vi "总氮固定站质控流程.vi"(6 "队列输入TN":refnum<queue>, 9 "总氮":bool, 10 "总氮量程切换":enum32{"H", "L", "AUTO"}(ring)=enum."AUTO") -> (3 "布尔":bool)   [LabVIEW 2016, in "质控单元.lvlib"]
panel:
  out "总氮中断报警":bool
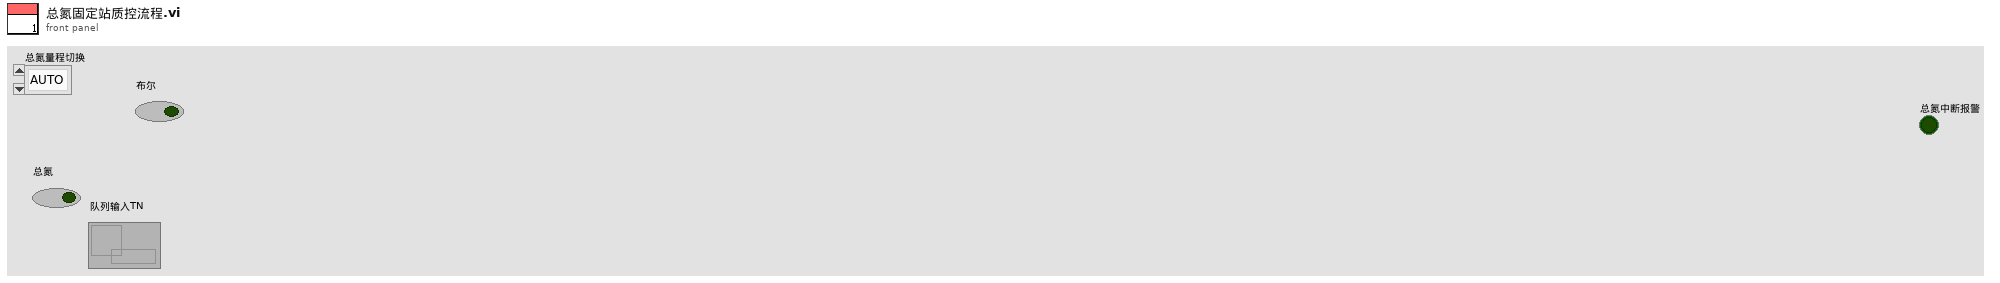
[diagram p1: front panel]
types:
  T1 = enum16{"待机", "启动氨氮水样", "氨氮测量中", "启动氨氮加标", "启动氨氮加标回收", "氨氮加标回收测量中", "启动总氮水样", "总氮测量中", "启动总氮加标", "启动总氮加标回收", "总氮加标回收测量中", "启动总磷水样", "总磷水样测量中", "启动总磷加标", "启动总磷加标回收", "总磷加标回收测量中", "结束"}
  T2 = cluster{"站号":u16, "量程切换":enum32{"H", "L", "AUTO"}, "控制命令":enum16{"启动测量", "标样核查", "零点核查", "跨度核查", "空白测试", "平行样测试", "加标回收", "空白校准", "标样校准", "初始化（清洗）", "停止测试", "仪器重启", "校时", "模式设置", "测量间隔设置"}, "模式设置":enum16{"待机", "连续模式", "周期模式", "定点模式", "受控模式", "手动模式"}, "测量间隔":u16}
  T3 = cluster{"时间标识":timestamp, "设备":string, "日志信息":string}
  T4 = cluster{"系统时间":timestamp, "工作状态":enum16{"空闲", "水样测试", "标样核查", "零点核查", "跨度核查", "空白测试", "平行样测试", "加标回收", "空白校准", "标样校准", "初始化（清洗）"}, "测量模式":enum16{"待机", "连续模式", "周期模式", "定点模式", "受控模式", "手动模式"}, "告警代码":enum16{"无告警", "缺试剂告警", "缺水样告警", "缺蒸馏水告警", "缺标液告警", "仪表漏液告警", "标定异常告警", "超量程告警", "加热异常", "低试剂预警", "超上限告警", "超下限告警", "仪表内部其他异常", "滴定异常告警", "电极异常告警", "量程切换告警", "参数设置告警", "PH电极电位异常", "电导率电极异常", "浊度光度异常", "溶解氧电极异常", "溶解氧光强异常", "温度异常告警", "PH异常告警", "溶解氧异常告警", "电导率异常告警", "浊度异常告警", "叶绿素异常告警", "藻密度异常告警", "蓝绿藻异常告警", "ORP异常告警", "氨氮异常告警", "清洁刷异常告警", "SD卡异常告警", "蓝牙异常告警", "Wifi异常告警", "流程异常告警"}, "故障代码":enum16{"无故障", "电机故障", "温度故障", "通讯故障", "滴定故障"}, "日志代码":u16, "软件版本":u16, "F0":sgl, "F1":sgl, "F2":sgl, "F3":sgl, "T":sgl, "H":sgl, "id":u16, "flowid":u16, "量程":u16, "总磷控温温度1":sgl, "营养盐控温温度2":sgl, "ADC":sgl}
  T5 = enum16{"空闲", "水样测试", "标样核查", "零点核查", "跨度核查", "空白测试", "平行样测试", "加标回收", "空白校准", "标样校准", "初始化（清洗）"}
  T6 = cluster{"因子编码":u32, "单位":u16, "标样参考值":sgl, "水样数据时间":timestamp, "水样实测值":sgl, "水样数据标识":string, "标样数据时间":timestamp, "标样实测值":sgl, "标样数据标识":string, "空白数据时间":timestamp, "空白实测值":sgl, "空白数据标识":string, "零点核查数据时间":timestamp, "零点核查实测值":sgl, "零点核查数据标识":string, "跨度核查数据时间":timestamp, "跨度核查实测值":sgl, "跨度核查数据标识":string, "加标回收数据时间":timestamp, "加标回收实测值":sgl, "加标回收数据标识":string, "平行样数据时间":timestamp, "平行样实测值":sgl, "平行样数据标识":string}
  T7 = cluster{"量程":dbl, "检出限":dbl, "加标前水样浓度":dbl, "加标后水样浓度":dbl, "加标水杯定容体积":dbl, "加标母液浓度":dbl, "加标体积":dbl, "加标回收率":dbl}
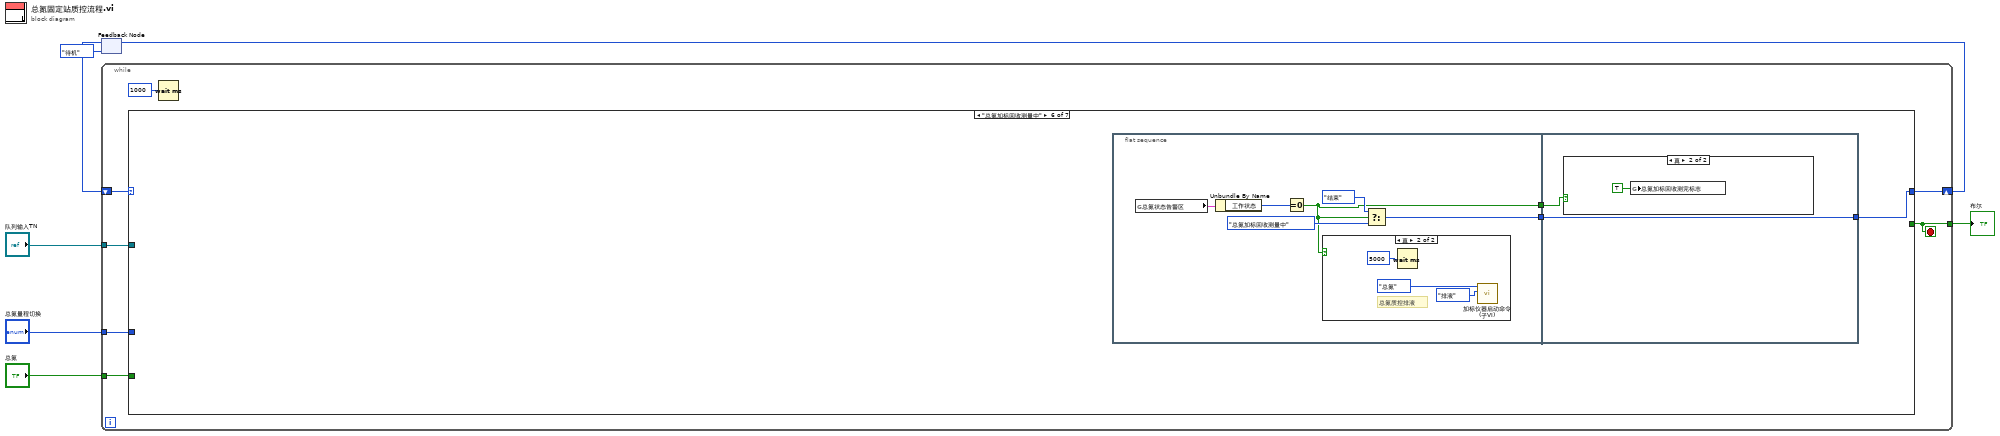
[diagram p0: block diagram]
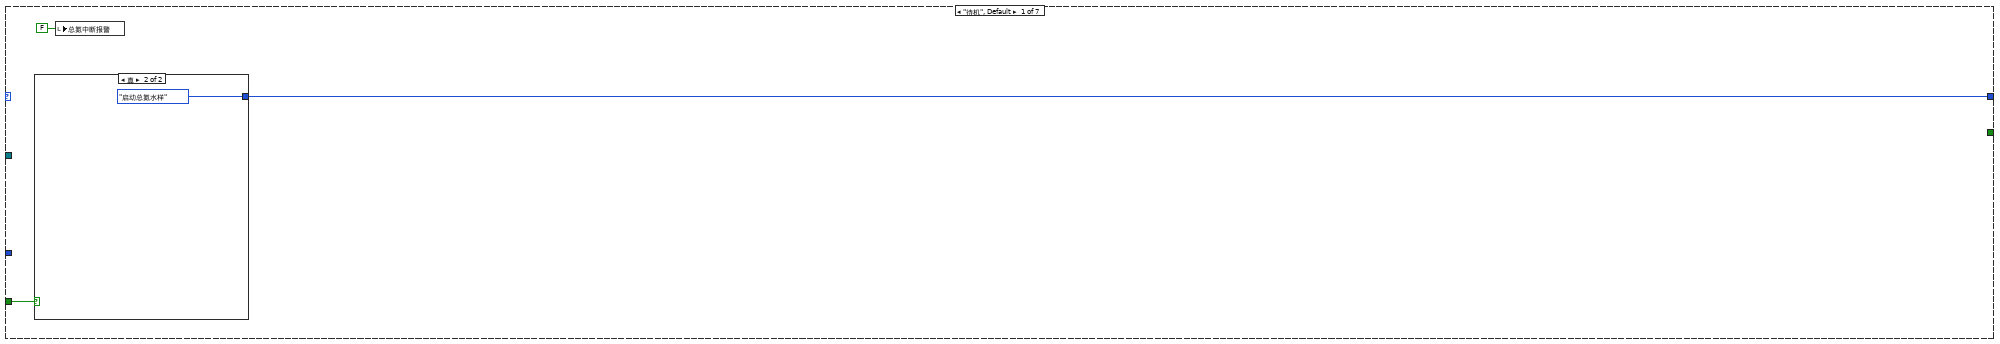
[diagram p2: hidden frame]
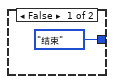
[diagram p3: hidden frame]
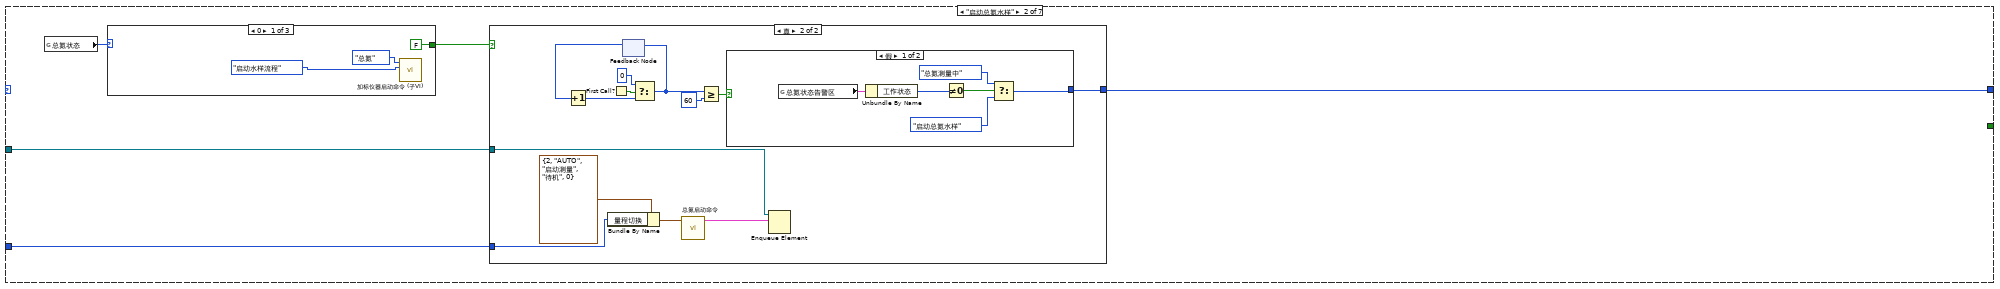
[diagram p4: hidden frame]
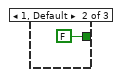
[diagram p5: hidden frame]
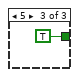
[diagram p6: hidden frame]
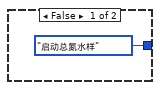
[diagram p7: hidden frame]
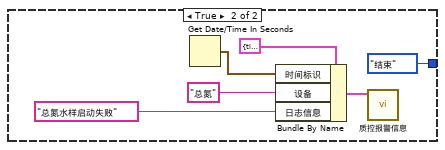
[diagram p8: hidden frame]
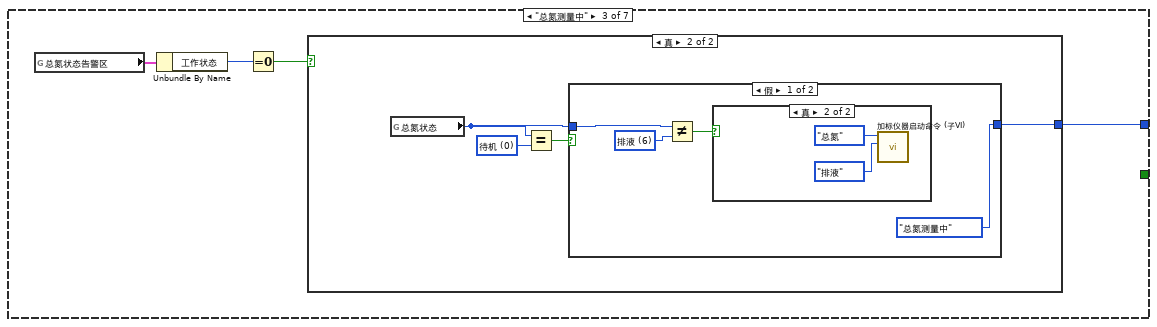
[diagram p9: hidden frame]
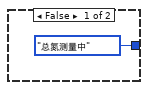
[diagram p10: hidden frame]
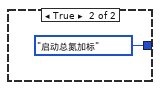
[diagram p12: hidden frame]
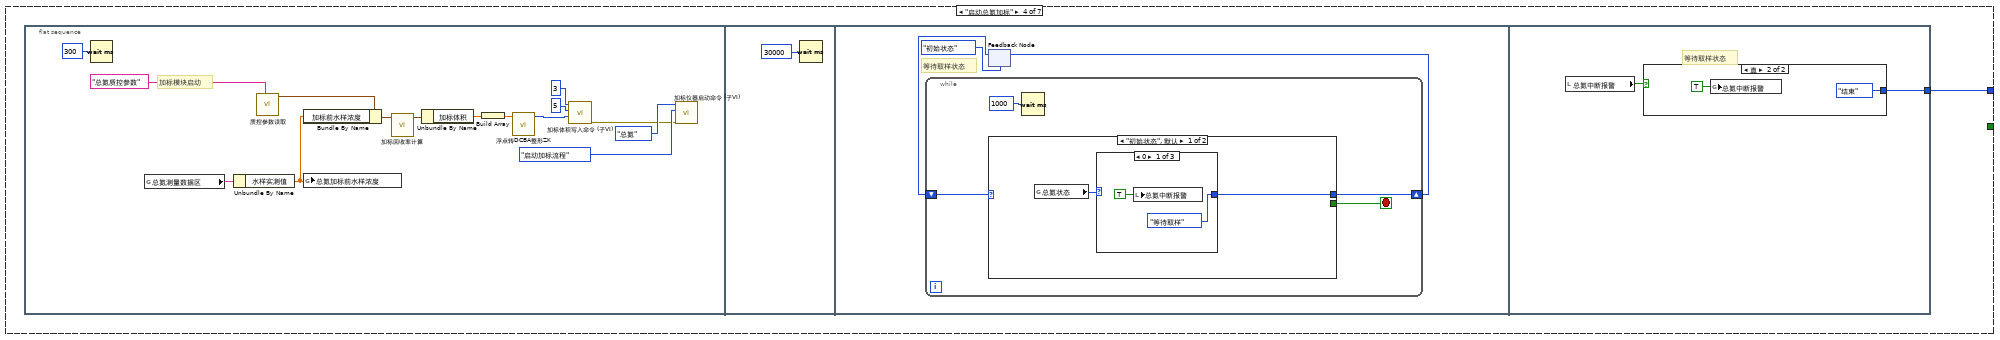
[diagram p13: hidden frame]
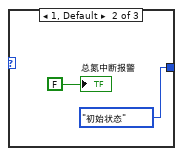
[diagram p14: hidden frame]
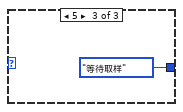
[diagram p15: hidden frame]
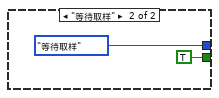
[diagram p16: hidden frame]
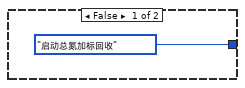
[diagram p17: hidden frame]
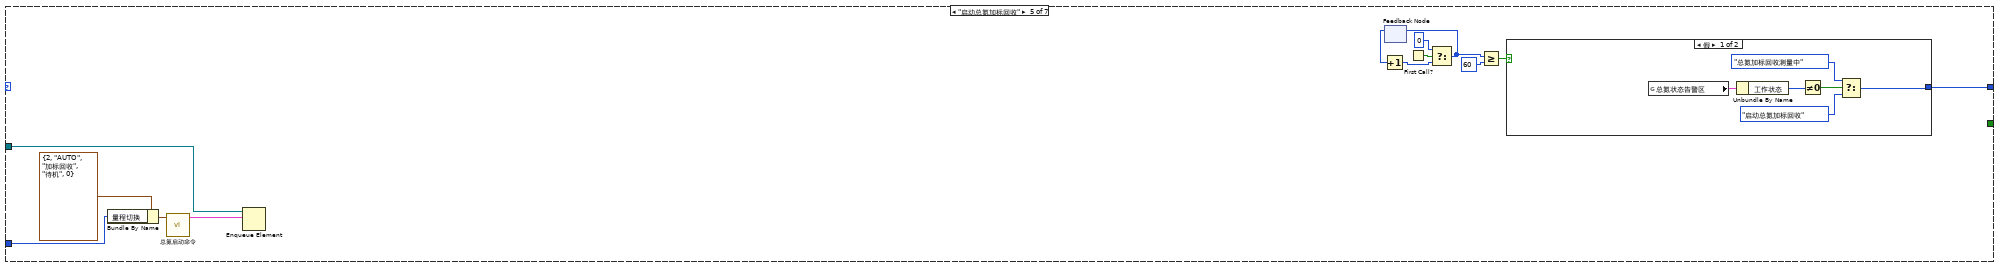
[diagram p18: hidden frame]
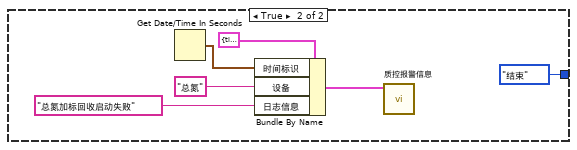
[diagram p19: hidden frame]
diagram:
  n1 = feedback #1(T1."待机") -> (w1:T1)
  n2 = while {
    tunnel: "队列输入TN" -> [w12]
    tunnel: "总氮量程切换" -> [w11]
    tunnel: "总氮" -> [w14]
    tunnel: [w8] -> w6
    shift-right: [w13] -> w4
    shift-left: w1 -> [w10]
    stop <- w8 stop-if-true
    n3 = case shown="\"总氮加标回收测量中\"" w10 {
      tunnel: [w17 w24 w56 w72 w115 w136 T1."结束"] -> w13
      tunnel: [_ _ _ _ _ _ TRUE] -> w8
      tunnel: w14 -> [w16 _ _ _ _ _ _]
      tunnel: w12 -> [_ w23 _ _ w114 _ _]
      tunnel: w11 -> [_ w22 _ _ w111 _ _]
      frame "待机", Default {
        n4 = case shown="真" w16 {
          tunnel: [T1."结束" T1."启动总氮水样"] -> w17
          frame False {
          }
          frame True {
          }
        }
        n5 = local write "总氮中断报警"(FALSE ("氨氮中断报警")) -> ()
      }
      frame "启动总氮水样" {
        n6 = global read "加标回收状态全局变量.vi" "总氮状态"() -> (w21:u16)
        n7 = case shown="0" w21 {
          tunnel: [FALSE ("s") FALSE ("s") TRUE ("s")] -> w20
          frame 0 {
            n8 = call "加标仪器启动命令 (子VI).vi"("启动命令"=enum16{"启动水样流程", "启动加标流程", "排液", "停止"}."启动水样流程", "仪器"=enum16{"", "氨氮", "总磷", "总氮", "CODMn", "CODCr"}."总氮") -> ()  [unwired: 9 in, 1 out]
          }
          frame 1, Default {
          }
          frame 5 {
          }
        }
        n9 = case shown="真" w20 {
          tunnel: [T1."启动总氮水样" w43] -> w24
          tunnel: w23 -> [_ w35]
          tunnel: w22 -> [_ w32]
          frame False {
          }
          frame True {
            n10 = Bundle By Name(cluster=T2 {"站号"=2, "量程切换"=enum."AUTO", "控制命令"=enum."启动测量", "模式设置"=enum."待机", "测量间隔"=0} ("参数"), "量程切换"=w32) -> (w34:T2)
            n11 = First Call?() -> (First Call?: T/F=w41:bool)
            n12 = feedback #2() -> (w40:i32)  [unwired: 1 in]
            n13 = Increment(x=w40) -> (x+1=w39:i32)
            n14 = Select(t=0, s=w41, f=w39) -> (s? t:f=w38:i32)
            n15 = feedback-in #2(w38) -> ()
            n16 = call "总氮启动命令.vi"("参数"=w34) -> ("启动命令"=w31:cluster{"命令":string, "data":variant})  [unwired: 10 in]
            n17 = Greater Or Equal?(x=w38, y=60) -> (x >= y?=w36:bool)
            n18 = case shown="假" w36 {
              tunnel: [w48 T1."结束"] -> w43
              frame False {
                n19 = global read "与总氮交互全局.vi" "总氮状态告警区"() -> (w45:T4)
                n20 = Unbundle By Name(w45) -> ("工作状态"=w44:T5)
                n21 = Not Equal To 0?(x=w44) -> (x != 0?=w49:bool)
                n22 = Select(t=T1."总氮测量中", s=w49, f=T1."启动总氮水样") -> (s? t:f=w48:T1)
              }
              frame True {
                n23 = Get Date/Time In Seconds() -> (seconds since 1Jan1904=w55:timestamp)
                n24 = Bundle By Name(cluster=T3 {"时间标识"=timestamp(0 s since 1904-01-01), "设备"="", "日志信息"=""} ("data in"), "时间标识"=w55, "设备"="总氮", "日志信息"="总氮水样启动失败") -> (w50:T3)
                n25 = call "质控报警信息.vi"("data in"=w50) -> ()  [unwired: 10 in, 1 out]
              }
            }
            n26 = Enqueue Element(queue=w35, element=w31) -> ()  [unwired: 2 in, 3 out]
          }
        }
      }
      frame "总氮测量中" {
        n27 = global read "与总氮交互全局.vi" "总氮状态告警区"() -> (w59:T4)
        n28 = Unbundle By Name(w59) -> ("工作状态"=w57:T5)
        n29 = Equal To 0?(x=w57) -> (x = 0?=w58:bool)
        n30 = case shown="真" w58 {
          tunnel: [T1."总氮测量中" w62] -> w56
          frame False {
          }
          frame True {
            w64 = u16 0 items=["待机", "润洗", "进样", "进样完成", "柱塞泵加标", "等待取液", "排液"] ("氨氮状态")
            n31 = global read "加标回收状态全局变量.vi" "总氮状态"() -> (w61:u16)
            n32 = Equal?(x=w61, y=w64) -> (x = y?=w63:bool)
            n33 = case shown="假" w63 {
              tunnel: [T1."总氮测量中" T1."启动总氮加标"] -> w62
              tunnel: w61 -> [w65 _]
              frame False {
                w67 = u16 6 items=["待机", "润洗", "进样", "进样完成", "柱塞泵加标", "等待取液", "排液"] ("氨氮状态")
                n34 = Not Equal?(x=w65, y=w67) -> (x != y?=w66:bool)
                n35 = case shown="真" w66 {
                  frame False {
                  }
                  frame True {
                    n36 = call "加标仪器启动命令 (子VI).vi"("启动命令"=enum16{"启动水样流程", "启动加标流程", "排液", "停止"}."排液", "仪器"=enum16{"", "氨氮", "总磷", "总氮", "CODMn", "CODCr"}."总氮") -> ()  [unwired: 9 in, 1 out]
                  }
                }
              }
              frame True {
              }
            }
          }
        }
      }
      frame "启动总氮加标" {
        n37 = flat-sequence {
          tunnel: [w106] -> w72
          frame #0 {
            # "加标模块启动"
            n38 = Wait (ms)(milliseconds to wait=u32 300 ("等待时间（毫秒）")) -> ()  [unwired: 1 out]
            n39 = global read "与总氮交互全局.vi" "总氮测量数据区"() -> (w80:T6)
            n40 = Unbundle By Name(w80) -> ("水样实测值"=w82:sgl)
            n41 = call "质控参数读取.vi"("section"="总氮质控参数") -> ("参数"=w85:T7)  [unwired: 9 in, 1 out]
            n42 = Bundle By Name(cluster=w85, "加标前水样浓度"=w82) -> (w86:T7)
            n43 = global write "水样浓度全局.vi" "总氮加标前水样浓度"(w82) -> ()
            n44 = call "加标回收率计算.vi"("参数"=w86) -> ("参数 out"=w84:T7)  [unwired: 9 in, 1 out]
            n45 = Unbundle By Name(w84) -> ("加标体积"=w83:dbl)
            n46 = Build Array(w83) -> (w79:dbl[])
            n47 = call "浮点转DCBA整形ZK.vi"("浮点数"=w79) -> ("DCBA整形输出"=w74:u16[])  [unwired: 10 in]
            n48 = call "加标体积写入命令 (子VI).vi"("values"=w74, "starting address"=u16 5, "Slave ID"=u16 3 ("value")) -> ("错误输出"=w73:errorcluster)  [unwired: 8 in]
            n49 = call "加标仪器启动命令 (子VI).vi"("错误输入（无错误）"=w73, "启动命令"=enum16{"启动水样流程", "启动加标流程", "排液", "停止"}."启动加标流程", "仪器"=enum16{"", "氨氮", "总磷", "总氮", "CODMn", "CODCr"}."总氮") -> ()  [unwired: 8 in, 1 out]
          }
          frame #1 {
            n50 = Wait (ms)(milliseconds to wait=u32 30000 ("等待时间（毫秒）")) -> ()  [unwired: 1 out]
          }
          frame #2 {
            # "等待取样状态"
            n51 = feedback #3(enum16{"初始状态", "等待取样"}."初始状态") -> (w90:enum16{"初始状态", "等待取样"})
            n52 = while {
              shift-right: [w94] -> w91
              shift-left: w90 -> [w95]
              stop <- w93 stop-if-true
              n53 = case shown="\"初始状态\", 默认" w95 {
                tunnel: [w97 enum16{"初始状态", "等待取样"}."等待取样"] -> w94
                tunnel: [_ TRUE] -> w93
                frame "初始状态", Default {
                  n54 = global read "加标回收状态全局变量.vi" "总氮状态"() -> (w96:u16)
                  n55 = case shown="0" w96 {
                    tunnel: [enum16{"初始状态", "等待取样"}."等待取样" enum16{"初始状态", "等待取样"}."初始状态" enum16{"初始状态", "等待取样"}."等待取样"] -> w97
                    frame 0 {
                      n56 = local write "总氮中断报警"(TRUE ("氨氮中断报警")) -> ()
                    }
                    frame 1, Default {
                      "总氮中断报警" <- FALSE ("总氮中断报警")
                    }
                    frame 5 {
                    }
                  }
                }
                frame "等待取样" {
                }
              }
              n57 = Wait (ms)(milliseconds to wait=u32 1000 ("等待时间（毫秒）")) -> ()  [unwired: 1 out]
            }
            n58 = feedback-in #3(w91) -> ()
          }
          frame #3 {
            # "等待取样状态"
            n59 = local read "总氮中断报警"() -> (w105:bool)
            n60 = case shown="真" w105 {
              tunnel: [T1."启动总氮加标回收" T1."结束"] -> w106
              frame False {
              }
              frame True {
                n61 = global write "质控中断报警全局.vi" "总氮中断报警"(TRUE ("总氮中断报警")) -> ()
              }
            }
          }
        }
      }
      frame "启动总氮加标回收" {
        n62 = Bundle By Name(cluster=T2 {"站号"=2, "量程切换"=enum."AUTO", "控制命令"=enum."加标回收", "模式设置"=enum."待机", "测量间隔"=0} ("参数"), "量程切换"=w111) -> (w113:T2)
        n63 = call "总氮启动命令.vi"("参数"=w113) -> ("启动命令"=w110:cluster{"命令":string, "data":variant})  [unwired: 10 in]
        n64 = Enqueue Element(queue=w114, element=w110) -> ()  [unwired: 2 in, 3 out]
        n65 = feedback #4() -> (w120:i32)  [unwired: 1 in]
        n66 = Increment(x=w120) -> (x+1=w119:i32)
        n67 = First Call?() -> (First Call?: T/F=w121:bool)
        n68 = Select(t=0, s=w121, f=w119) -> (s? t:f=w118:i32)
        n69 = feedback-in #4(w118) -> ()
        n70 = Greater Or Equal?(x=w118, y=60) -> (x >= y?=w116:bool)
        n71 = case shown="假" w116 {
          tunnel: [w126 T1."结束"] -> w115
          frame False {
            n72 = global read "与总氮交互全局.vi" "总氮状态告警区"() -> (w123:T4)
            n73 = Unbundle By Name(w123) -> ("工作状态"=w128:T5)
            n74 = Not Equal To 0?(x=w128) -> (x != 0?=w127:bool)
            n75 = Select(t=T1."总氮加标回收测量中", s=w127, f=T1."启动总氮加标回收") -> (s? t:f=w126:T1)
          }
          frame True {
            n76 = Get Date/Time In Seconds() -> (seconds since 1Jan1904=w134:timestamp)
            n77 = Bundle By Name(cluster=T3 {"时间标识"=timestamp(0 s since 1904-01-01), "设备"="", "日志信息"=""} ("data in"), "时间标识"=w134, "设备"="总氮", "日志信息"="总氮加标回收启动失败") -> (w129:T3)
            n78 = call "质控报警信息.vi"("data in"=w129) -> ()  [unwired: 10 in, 1 out]
          }
        }
      }
      frame "总氮加标回收测量中" {
        n79 = flat-sequence {
          tunnel: [w142] -> w137
          tunnel: [w138] -> w135
          tunnel: [w148] -> w136
          tunnel: w137 -> [w148]
          tunnel: w135 -> [w147]
          frame #0 {
            n80 = global read "与总氮交互全局.vi" "总氮状态告警区"() -> (w139:T4)
            n81 = Unbundle By Name(w139) -> ("工作状态"=w143:T5)
            n82 = Equal To 0?(x=w143) -> (x = 0?=w138:bool)
            n83 = case shown="真" w138 {
              frame False {
              }
              frame True {
                # "总氮质控排液"
                n84 = Wait (ms)(milliseconds to wait=u32 5000 ("等待时间（毫秒）")) -> ()  [unwired: 1 out]
                n85 = call "加标仪器启动命令 (子VI).vi"("启动命令"=enum16{"启动水样流程", "启动加标流程", "排液", "停止"}."排液", "仪器"=enum16{"", "氨氮", "总磷", "总氮", "CODMn", "CODCr"}."总氮") -> ()  [unwired: 9 in, 1 out]
              }
            }
            n86 = Select(t=T1."结束", s=w138, f=T1."总氮加标回收测量中") -> (s? t:f=w142:T1)
          }
          frame #1 {
            n87 = case shown="真" w147 {
              frame False {
              }
              frame True {
                n88 = global write "质控测完标志全局 1.vi" "总氮加标回收测完标志"(TRUE) -> ()
              }
            }
          }
        }
      }
      frame "结束" {
        n89 = Wait (ms)(milliseconds to wait=u32 5000 ("等待时间（毫秒）")) -> ()  [unwired: 1 out]
      }
    }
    n90 = Wait (ms)(milliseconds to wait=u32 1000 ("等待时间（毫秒）")) -> ()  [unwired: 1 out]
  }
  "布尔" <- w6
  n91 = feedback-in #1(w4) -> ()
